vi "PV ActiveLine - Error Status.vi"(8 "Fehler (Eingang)":errorcluster, 11 "Referenz in":refnum<visa-resource-name>) -> (0 "Cluster (Ausgang)":errorcluster, 1 "Errortext":string, 2 "Errornumber":u16, 3 "Referenz out":refnum<visa-resource-name>)   [LabVIEW 2013, in "PV ActiveLine.lvlib"]
doc: "ERR - Error Status\n\nReceive: aaaa\n\nError status,\naaaa =\n0000 –> No error\n1000 –> ERROR (controller error (see display on front panel)\n0100 –> NO HWR (no hardware)\n0010 –> PAR (inadmissible parameter)\n0001 –> SYN (Syntax error)\n\nThe ERROR word is cancelled when read out. If the error persists, it is immediately set again."
uses:
  <instrlib>/PV ActiveLine/PV ActiveLine.lvlib
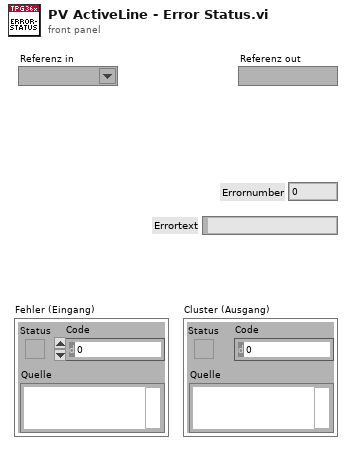
[diagram p1: front panel]
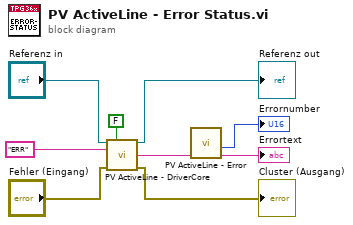
[diagram p0: block diagram]
diagram:
  n1 = call <instrlib>:"PV ActiveLine - DriverCore.vi"("Referenz in"="Referenz in", "Write/Read"=FALSE, "Command"="ERR", "Fehler (Eingang)"="Fehler (Eingang)") -> ("Referenz out"=→"Referenz out":refnum<visa-resource-name>, "String Out"=w6:string, "Cluster (Ausgang)"=→"Cluster (Ausgang)":errorcluster)  [unwired: 9 in]
  n2 = call <instrlib>:"PV ActiveLine - Error.vi"("String IN"=w6) -> ("Errortext"=→"Errortext":string, "Errornumber"=→"Errornumber":i32)  [unwired: 8 in]
